vi "AB_Generate_Error_Cluster.vi"(8 "error in (no error)":errorcluster, 9 "Additional Message":string, 10 "source":string, 11 "Code":i32(ring) items=["No error", "Argument error", "Memory is full", "Out of zone", "End of file", "File already open", "Generic file I/O error", "File not found", "File permission error", "Disk is full", "Duplicate path", "Too many files open", "System feature not enabled", "Resource file not found", "Cannot add resource", "Resource not found", "Image not found", "Image memory error", "Pen does not exist", "Config type invalid", "Config token not found", "Config parse error", "Config memory error", "Bad external code format", "Bad external code offset", "External code not present", "Null window", "Destroy window error", "Null menu", "Print aborted", "Bad print record", "Print driver error", "Windows error during printing", "Memory error during printing", "Print dialog error", "Generic print error", "Invalid device refnum", "Device not found", "Device parameter error", "Device unit error", "Cannot open device", "Device call aborted", "Generic error", "Cancelled by user", "Object ID too low", "Object ID too high", "Object not in heap", "Unknown heap", "Unknown object (invalid DefProc)", "Unknown object (DefProc not in table)", "Message out of range", "Invalid (null) method", "Unknown message", "Manager call not supported", "Bad address", "Network operation in progress", "Network operation timed out", "Connection is busy", "Network attribute not supported", "Network error", "Address in use", "System out of memory", "Connection aborted", "Connection refused", "Not connected", "Already connected", "Connection closed", "Initialization error (interapplication manager)", "Bad occurrence", "Wait on unbound occurrence handler", "Occurrence queue overflow", "Datalog type conflict", "Unused", "Unrecognized type (interapplication manager)", "Memory corrupt", "Failed to make temporary DLL", "Old CIN version", "Drag socket not found", "Failed to load drop-object", "Failed to register OLE object", "Failed to release OLE object", "Format specifier type mismatch", "Unknown format specifier", "Too few format specifiers", "Too many format specifiers", "Scan failed", "Newer CIN version", "Error converting to variant", "Runtime menu error", "Password tampered", "Variant attribute not found", "Incompatible variant data type", "Event data is not available", "Event Store is not present", "Occurrence is not found", "Event Queue is not created", "Event info is not available in the type library", "Refnum passed is NULL", "Error retrieving Class GUID", "Error retrieving CoClass GUID", "Error retrieving TypeLib GUID.", "Bad built application magic bytes.", "Specific driver is different from the specific driver associated with the Logical Name.", "There is no session opened to the class driver.", "Max Error", "MAX - Error with config objects", "MAX - Error loading configuration", "MAX - Group not supported", "Singlecast connections can not send to multicast addresses.", "Multicast connections can not send to singlecast addresses.", "Specified IP address not in multicast address range.", "Attempt to write to read-only multicast connection.", "Attempt to read from write-only multicast connection.", "The buffer used to receive a datagram was smaller than the datagram itself"]) -> (0 "error out":errorcluster)   [LabVIEW 2020]
uses:
  <vilib>/Utility/error.llb/DialogType.ctl
  <resource>/Framework/Providers/Common/provcom_StringGlobals.vi
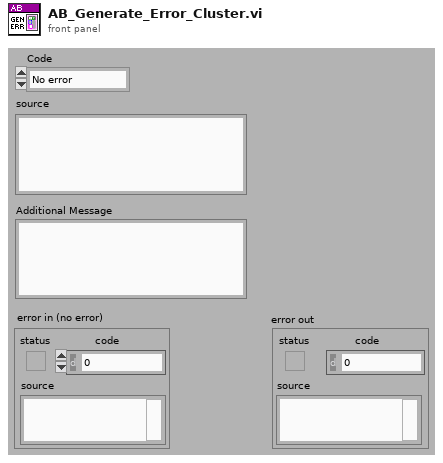
[diagram p1: front panel]
types:
  T1 = typedef "DialogType.ctl" = u16
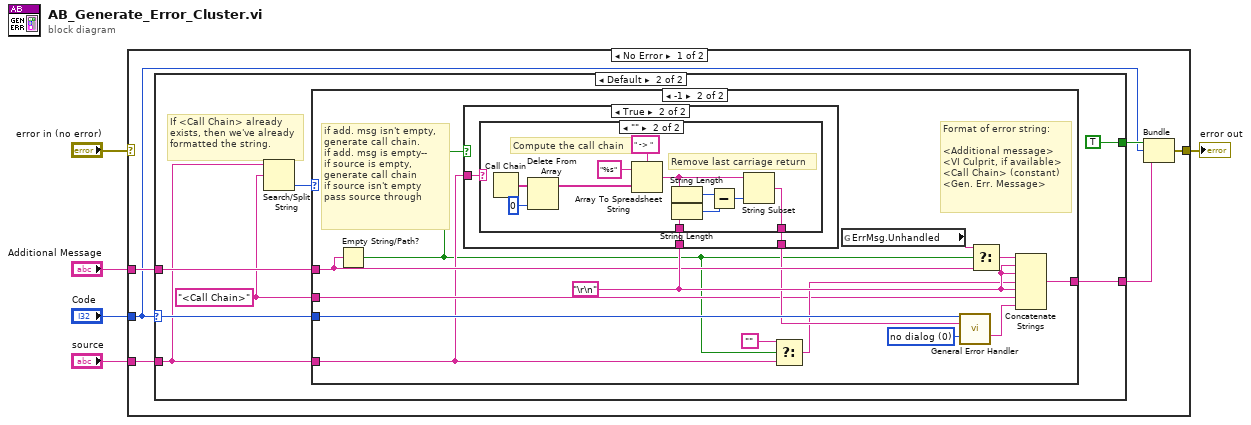
[diagram p0: block diagram]
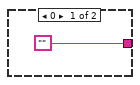
[diagram p2: hidden frame]
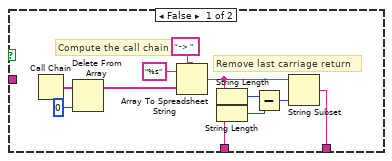
[diagram p4: hidden frame]
diagram:
  n1 = case shown="No Error" "error in (no error)" {
    selector: "error in (no error)" -> [_ w61]
    tunnel: [w11 w61] -> w5
    tunnel: "Additional Message" -> [w8 _]
    tunnel: "source" -> [w7 _]
    tunnel: "Code" -> [w6 _]
    frame No Error {
      n2 = case shown="Default" w6 {
        selector: w6 -> [_ w17]
        tunnel: [_ TRUE] -> w10
        tunnel: ["" w19] -> w9
        tunnel: w8 -> [_ w16]
        tunnel: w7 -> [_ w14]
        frame 0 {
        }
        frame Default {
          w15 = "<Call Chain>" ("string")
          # "If <Call Chain> already\nexists, then we've already\nformatted the string."
          n3 = Search/Split String(string=w14, search string/char (-)=w15) -> (offset of match=w13:i32)  [unwired: 3 out]
          n4 = case shown="-1" w13 {
            tunnel: [w20 w34] -> w19
            tunnel: w17 -> [_ w32]
            tunnel: w16 -> [_ w27]
            tunnel: w14 -> [w20 w22]
            tunnel: w15 -> [_ w23]
            frame Default {
            }
            frame -1 {
              w31 = T1 0 items=["no dialog", "OK message", "continue or stop message", "OK message + warnings", "continue/stop + warnings"] ("type of dialog (OK msg:1)")
              w33 = "\r\n"
              # "if add. msg isn't empty,\ngenerate call chain.\nif add. msg is empty--\nif source is empty,\ngenerate call chain\nif source isn't empty\npass source through"
              # "Format of error string:\n\n<Additional message>\n<VI Culprit, if available>\n<Call Chain> (constant)\n<Gen. Err. Message>"
              n5 = Empty String/Path?(string/path=w27) -> (empty?=w21:bool)
              n6 = case shown="True" w21 {
                tunnel: w33 -> [w36 w48]
                tunnel: [w37 w47] -> w26
                tunnel: w22 -> [_ w46]
                frame False {
                  # "Remove last carriage return"
                  # "Compute the call chain"
                  n7 = Call Chain() -> (call chain=w43:string[])
                  n8 = Delete From Array(array=w43, index=0 ("Index")) -> (array with subset deleted=w35:string[])  [unwired: 1 in, 1 out]
                  n9 = Array To Spreadsheet String(delimiter (Tab)=" -> ", array=w35, 3:"%s" ("format string")) -> (spreadsheet string=w39:string)
                  n10 = String Length(string=w39) -> (length=w41:i32)
                  n11 = String Length(string=w36) -> (length=w38:i32)
                  n12 = Subtract(x=w41, y=w38) -> (x-y=w42:i32)
                  n13 = String Subset(string=w39, length (rest)=w42) -> (substring=w37:string)  [unwired: 1 out]
                }
                frame True {
                  n14 = case shown="\"\"" w46 {
                    selector: w46 -> [w49 _]
                    tunnel: w48 -> [_ w60]
                    tunnel: [w49 w59] -> w47
                    frame Default {
                    }
                    frame "" {
                      # "Remove last carriage return"
                      # "Compute the call chain"
                      n15 = Call Chain() -> (call chain=w56:string[])
                      n16 = Delete From Array(array=w56, index=0 ("Index")) -> (array with subset deleted=w50:string[])  [unwired: 1 in, 1 out]
                      n17 = Array To Spreadsheet String(delimiter (Tab)=" -> ", array=w50, 3:"%s" ("format string")) -> (spreadsheet string=w52:string)
                      n18 = String Length(string=w52) -> (length=w54:i32)
                      n19 = String Length(string=w60) -> (length=w51:i32)
                      n20 = Subtract(x=w54, y=w51) -> (x-y=w55:i32)
                      n21 = String Subset(string=w52, length (rest)=w55) -> (substring=w59:string)  [unwired: 1 out]
                    }
                  }
                }
              }
              n22 = Select(t="", s=w21, f=w22) -> (s? t:f=w24:string)
              n23 = global read "provcom_StringGlobals.vi" "ErrMsg.Unhandled"() -> (w28:string)
              n24 = call <vilib>:"General Error Handler.vi"("[error code] (0)"=w32, "[error source] (\" \")"=w26, "type of dialog (OK msg:1)"=w31) -> ("message"=w30:string)  [unwired: 2 in, 10 out]
              n25 = Select(t=w28, s=w21, f=w27) -> (s? t:f=w29:string)
              n26 = Concatenate Strings(w29, w33, w33, w24, w33, w23, w30) -> (w34:string)
            }
          }
        }
      }
      n27 = Bundle(w10, "Code"=w6, "source"=w9) -> (w11:cluster{bool, "Code":i32, "source":string})  [unwired: 1 out]
    }
    frame Error {
    }
  }
  "error out" <- w5
